vi "oa_TV Update Angle interval (1Chan).vi"(5 "reset? (F)":bool, 8 "error in (no error)":errorcluster, 9 "pulse/revolution":i32=1, 10 "revulotion index":i32, 11 "pulse positions":dbl[](array[numeric])) -> (0 "error out":errorcluster, 3 "angle intervals":dbl[](array[numeric]))   [LabVIEW 2017, in "SoundVib_Torsional.lvlib"]
uses:
  <vilib>/addons/Sound and Vibration/Order Analysis/Torsional Vibration/SoundVib_Torsional.lvlib
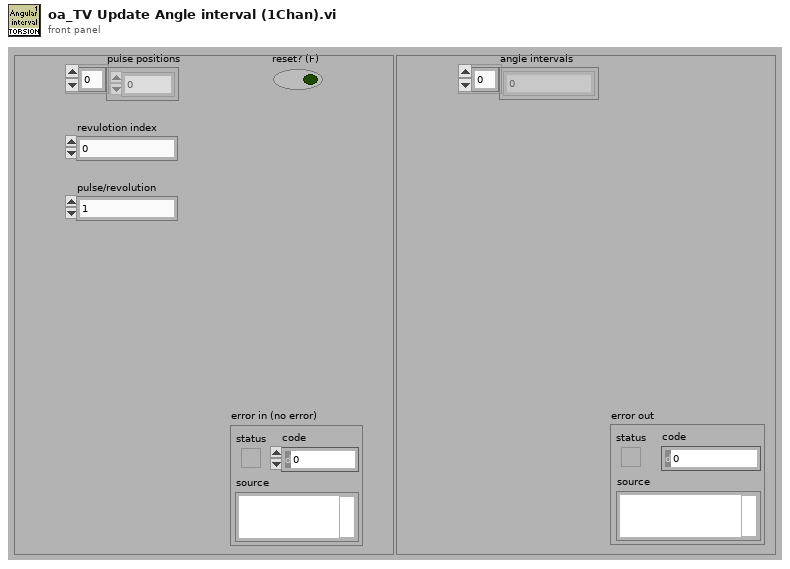
[diagram p1: front panel]
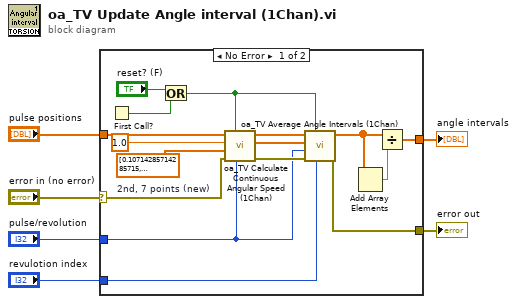
[diagram p0: block diagram]
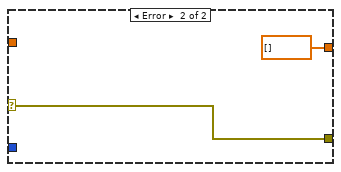
[diagram p2: hidden frame]
diagram:
  n1 = case shown="No Error" "error in (no error)" {
    selector: "error in (no error)" -> [w12 w24]
    tunnel: "pulse/revolution" -> [w8 _]
    tunnel: "pulse positions" -> [w14 _]
    tunnel: "revulotion index" -> [w18 _]
    tunnel: [w20 dbl[] []] -> w1
    tunnel: [w17 w24] -> w2
    frame No Error {
      w13 = dbl[] [0.10714285714285715, 0.07142857142857142, 0.035714285714285705, -1.5209319782164736e-17, -0.03571428571428571, -0.07142857142857142, -0.10714285714285715]  # 2nd, 7 points (new)
      n2 = First Call?() -> (First Call?: T/F=w21:bool)
      n3 = Or(x="reset? (F)", y=w21) -> (x .or. y?=w15:bool)
      n4 = call <vilib>:"oa_TV Calculate Continuous Angular Speed (1Chan).vi"("pulse/revolution (1)"=w8, "reset? (False)"=w15, "error in (no error)"=w12, "filter coefficients"=w13, "deltaX"=1.0, "Y[n]"=w14) -> ("error out"=w11:errorcluster, "dY[n]/dX[n]"=w9:dbl[], "pulse out"=w10:dbl[])  [unwired: 3 in]
      n5 = call <vilib>:"oa_TV Average Angle Intervals (1Chan).vi"("revulotion index"=w18, "reset? (F)"=w15, "error in (no error)"=w11, "pulse/revolution"=w8, "RPM"=w9, "time index"=w10) -> ("error out"=w17:errorcluster, "angle intervals"=w16:dbl[])  [unwired: 4 in]
      n6 = Add Array Elements(numeric array=w16) -> (sum=w19:dbl)
      n7 = Divide(x=w16, y=w19) -> (x/y=w20:dbl[])
    }
    frame Error {
    }
  }
  "angle intervals" <- w1
  "error out" <- w2
